vi "Create AO Channel.vi"(6 "units":string, 8 "error in":errorcluster, 9 "index":i32, 10 "default value":dbl, 11 "name":string) -> (0 "error out":errorcluster, 3 "AO channel out":refnum<class "AO Channel.lvclass">)   [LabVIEW 2017, in "AO Channel.lvclass"]
uses:
  AO Channel.lvclass
  Desktop/Scan Engine Sandbox/Channel Classes/Channel/Type.ctl
  Desktop/Scan Engine Sandbox/Channel Classes/Channel/Channel.lvclass
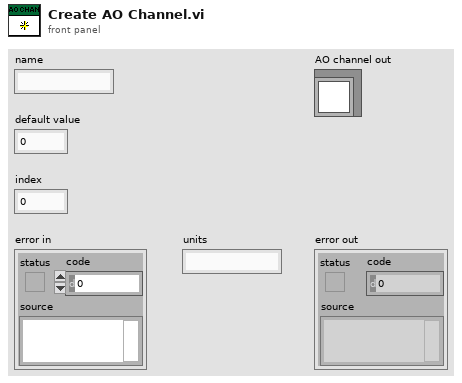
[diagram p1: front panel]
types:
  T1 = typedef "Channel.lvclass/Type.ctl" = enum16{"Input", "Output"}
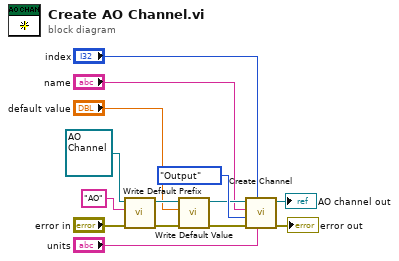
[diagram p0: block diagram]
diagram:
  n1 = call-dynamic "Write Default Prefix.vi"("error in"="error in", "default prefix"="AO" ("Default Prefix"), "channel in"=refnum<class "AO Channel.lvclass"> refnum ("AO Channel.lvclass")) -> ("error out"=w11:errorcluster, "channel out"=w12:refnum<class "AO Channel.lvclass">)  [unwired: 7 in]
  n2 = call-dynamic "Write Default Value.vi"("error in"=w11, "default value"="default value", "analog channel in"=w12) -> ("error out"=w10:errorcluster, "analog channel out"=w9:refnum<class "AO Channel.lvclass">)  [unwired: 7 in]
  n3 = call-dynamic "Create Channel.vi"("units"="units", "index"="index", "error in"=w10, "type"=Type."Output", "name"="name", "channel in"=w9) -> ("error out"=→"error out":errorcluster, "channel out"=→"AO channel out":refnum<class "AO Channel.lvclass">)  [unwired: 4 in]
